vi "Register Show Dialog to Settings Model.vi"(8 "error in (no error)":errorcluster, 11 "UI Controller in":refnum<class "UI Controller.lvclass">) -> (0 "error out":errorcluster, 3 "UI Controller out":refnum<class "UI Controller.lvclass">)   [LabVIEW 2015, in "UI Controller.lvlib" / "UI Controller.lvclass"]
uses:
  UI Controller.lvclass
  Models/Settings Model/Settings Model Messages/Concrete Show Dialog Msg/Concrete Show Dialog Msg.lvclass
  Views/Settings View/Settings View Messages/Register Show Dialog/Register Show Dialog.lvclass
  <vilib>/ActorFramework/Message Enqueuer/Message Enqueuer.lvclass/Message Enqueuer.ctl
  <vilib>/ActorFramework/Message Priority Queue/Priority Enqueue.vi
  <vilib>/ActorFrameworkMVC/Abstract Controller/Abstract Controller/Abstract Controller.lvclass
  <vilib>/ActorFramework/Message Enqueuer/Message Enqueuer.lvclass
panel:
  # "NOTICE -- YOU MUST LEAVE THIS NOTICE IN PLACE.\n\nCopyright (c) 2015, LIANG LIU Shawn.Liu.cn@gmail.com\nAll rights reserved.\n\nRedistribution and use in source and binary forms, with or without modification, are permitted provided that the following conditions are met:\n-Redistributions of source code must retain the above copyright notice, this list of conditions and the following disclaimer.\n-Redistributions in binary form must reproduce the above copyright notice, this list of conditions and the following disclaimer in the documentation and/or other materials provided with the distribution.\n-Neither the name of the eLp nor the names of its contributors may be used to endorse or promote products derived from this software without specific prior written permission.\n\nTHIS SOFTWARE IS PROVIDED BY THE COPYRIGHT HOLDERS AND CONTRIBUTORS \"AS IS\" AND ANY EXPRESS OR IMPLIED WARRANTIES, INCLUDING, BUT NOT LIMITED TO, THE IMPLIED WARRANTIES OF MERCHANTABILITY AND FITNESS FOR A PARTICULAR PURPOSE ARE DISCLAIMED. IN NO EVENT SHALL THE COPYRIGHT HOLDER OR CONTRIBUTORS BE LIABLE FOR ANY DIRECT, INDIRECT, INCIDENTAL, SPECIAL, EXEMPLARY, OR CONSEQUENTIAL DAMAGES (INCLUDING, BUT NOT LIMITED TO, PROCUREMENT OF SUBSTITUTE GOODS OR SERVICES; LOSS OF USE, DATA, OR PROFITS; OR BUSINESS INTERRUPTION) HOWEVER CAUSED AND ON ANY THEORY OF LIABILITY, WHETHER IN CONTRACT, STRICT LIABILITY, OR TORT (INCLUDING NEGLIGENCE OR OTHERWISE) ARISING IN ANY WAY OUT OF THE USE OF THIS SOFTWARE, EVEN IF ADVISED OF THE POSSIBILITY OF SUCH DAMAGE."
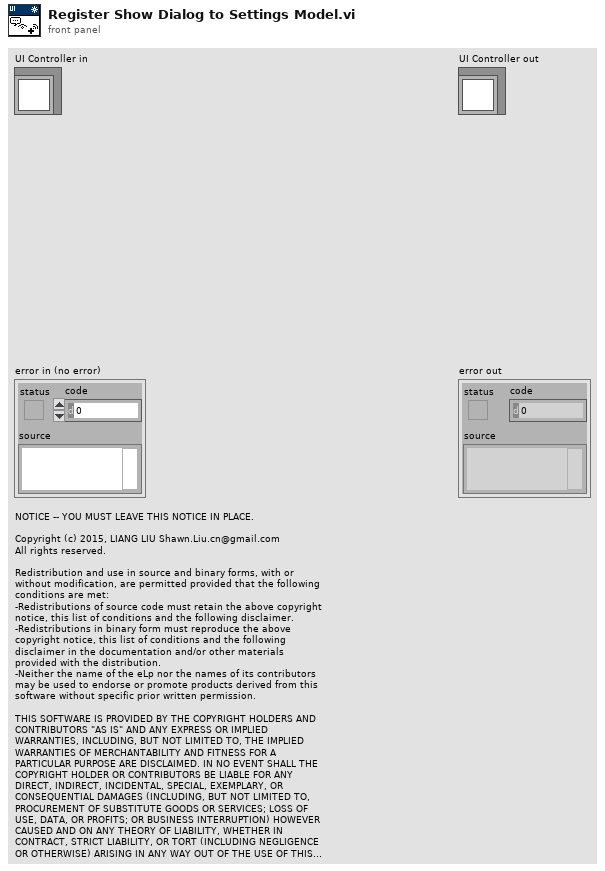
[diagram p1: front panel]
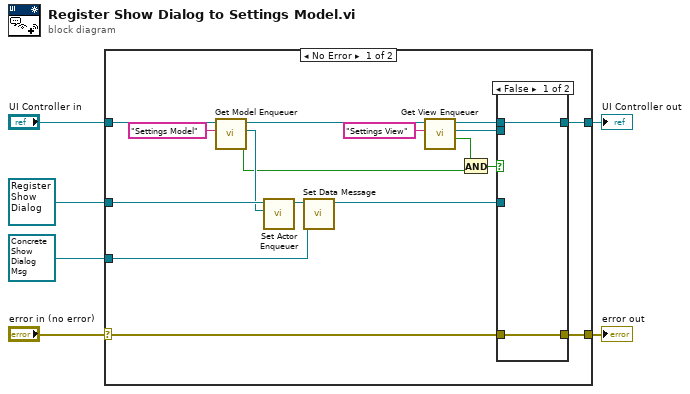
[diagram p0: block diagram]
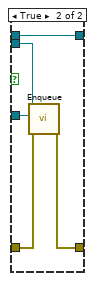
[diagram p2: hidden frame]
diagram:
  n1 = case shown="No Error" "error in (no error)" {
    selector: "error in (no error)" -> [w21 w32]
    tunnel: "UI Controller in" -> [w23 w31]
    tunnel: [w22 w32] -> w5
    tunnel: refnum<class "Register Show Dialog.lvclass"> refnum ("Settings Flyout.lvlib:Register Show Dialog.lvclass") -> [w20 _]
    tunnel: [w19 w31] -> w2
    tunnel: refnum<class "Concrete Show Dialog Msg.lvclass"> refnum ("Settings Model.lvlib:Concrete Show Dialog Msg.lvclass") -> [w18 _]
    frame No Error {
      n2 = call <vilib>:"Get Model Enqueuer.vi"("Model Name"="Settings Model", "Abstract Controller in"=w23) -> ("Found?"=w9:bool, "Model Enqueuer"=w15:refnum<class "Message Enqueuer.lvclass">, "Abstract Controller out"=w13:refnum<class "UI Controller.lvclass">)  [unwired: 6 in, 1 out]
      n3 = call-dynamic "Set Actor Enqueuer.vi"("Actor Enqueuer"=w15, "Registration Message in"=w20) -> ("Registration Message out"=w16:refnum<class "Register Show Dialog.lvclass">)  [unwired: 9 in]
      n4 = call-dynamic "Set Data Message.vi"("Data Message"=w18, "Registration Message in"=w16) -> ("Registration Message out"=w14:refnum<class "Register Show Dialog.lvclass">)  [unwired: 9 in]
      n5 = call <vilib>:"Get View Enqueuer.vi"("View Name"="Settings View" ("Model Name"), "Abstract Controller in"=w13) -> ("Found?"=w8:bool, "View Enqueuer"=w11:refnum<class "Message Enqueuer.lvclass">, "Abstract Controller out"=w12:refnum<class "UI Controller.lvclass">)  [unwired: 6 in, 1 out]
      n6 = And(x=w8, y=w9) -> (x .and. y?=w7:bool)
      n7 = case shown="False" w7 {
        tunnel: w14 -> [_ w30]
        tunnel: w12 -> [w25 w29]
        tunnel: [w25 w29] -> w19
        tunnel: w21 -> [w24 w28]
        tunnel: [w24 w27] -> w22
        tunnel: w11 -> [_ w26]
        frame False {
        }
        frame True {
          n8 = call <vilib>:"Enqueue.vi"("error in (no error)"=w28, "Message"=w30, "Message Enqueuer in"=w26) -> ("error out"=w27:errorcluster)  [unwired: 7 in, 1 out]
        }
      }
    }
    frame Error {
    }
  }
  "error out" <- w5
  "UI Controller out" <- w2
